vi "write eight strings to csv line and file.vi"(0 "Path":path, 1 "item 3":string, 2 "item 2":string, 3 "item 1":string, 5 "item 4":string, 7 "item 5":string, 9 "item 6":string, 11 "error in (no error)":errorcluster, 12 "item 7":string, 13 "item 8":string) -> (4 "csv string":string, 15 "error out":errorcluster)   [LabVIEW 2013]
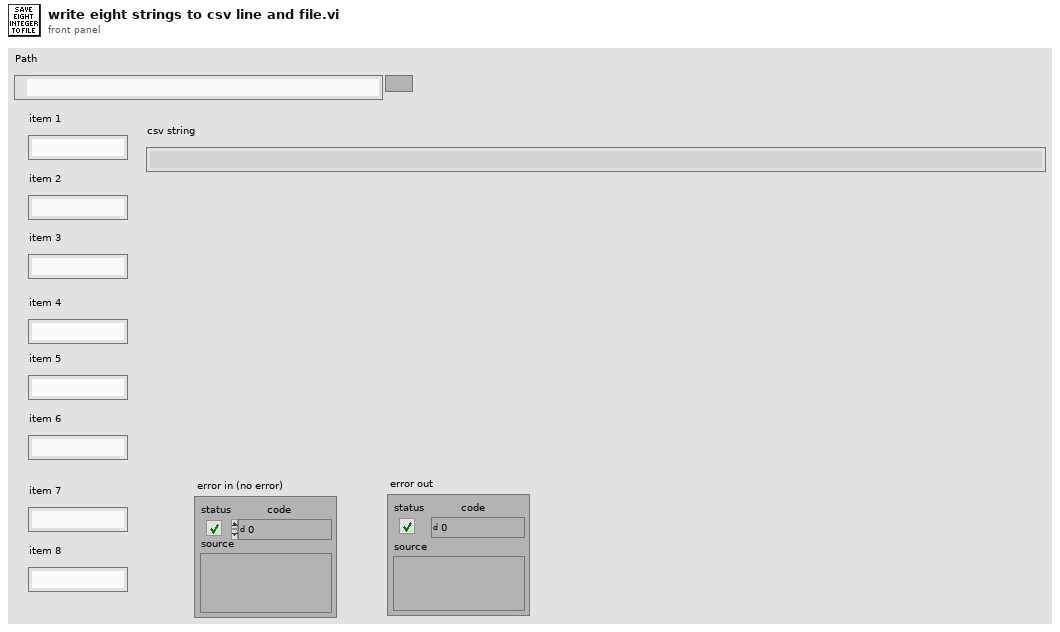
[diagram p1: front panel]
types:
  T1 = enum16{"open", "replace", "create", "open or create", "replace or create", "replace or create with confirmation"}
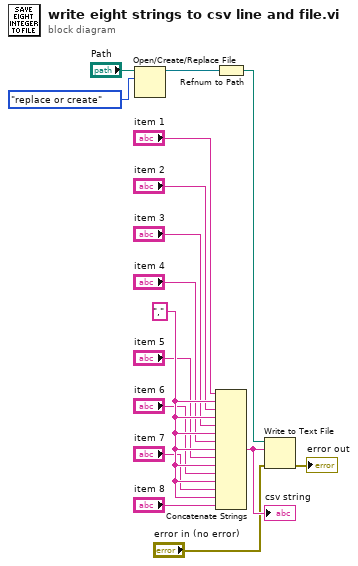
[diagram p0: block diagram]
diagram:
  w13 = "," ("element")
  n1 = Open/Create/Replace File(file path (use dialog)="Path", operation (0:open)=T1."replace or create") -> (refnum out=w16:refnum<file>)  [unwired: 4 in, 2 out]
  n2 = Refnum to Path(1:w16) -> (0:w12:path)
  n3 = Concatenate Strings("item 1", w13, "item 2", w13, "item 3", w13, "item 4", w13, "item 5", w13, "item 6", w13, "item 7", w13, "item 8") -> (w11:string)
  "csv string" <- w11
  n4 = Write to Text File(file (use dialog)=w12, text=w11, error in="error in (no error)") -> (error out=→"error out":errorcluster)  [unwired: 1 in, 2 out]
